vi "ReadNumeric.vi"(1 "reference":refnum<vi>) -> (0 "Numeric":T10)   [LabVIEW 2013]
uses:
  <vilib>/Utility/miscctls.llb/LVBoundsTypeDef.ctl
  <vilib>/Utility/miscctls.llb/LVPositionTypeDef.ctl
  <vilib>/Utility/miscctls.llb/LVRectTypeDef.ctl
  <vilib>/Utility/miscctls.llb/LVDataSocketStatusTypeDef.ctl
  <vilib>/Utility/miscctls.llb/LVKeyNavTypeDef.ctl
  <vilib>/Utility/miscctls.llb/LVMinMaxIncTypeDef.ctl
  <vilib>/Utility/miscctls.llb/LVKeyTypeDef.ctl
  <vilib>/numeric/LVNumericRepresentation.ctl
  <vilib>/Utility/miscctls.llb/LVOutOfRangeActionTypeDef.ctl
panel:
  out "error out 77":errorcluster
  out "error out 76":errorcluster
  out "error out 75":errorcluster
  out "error out 74":errorcluster
  out "error out 73":errorcluster
  out "error out 72":errorcluster
  out "error out 71":errorcluster
  out "error out 70":errorcluster
  out "error out 69":errorcluster
  out "error out 68":errorcluster
  out "error out 67":errorcluster
  out "error out 66":errorcluster
  out "error out 65":errorcluster
  out "error out 64":errorcluster
  out "error out 63":errorcluster
  out "error out 62":errorcluster
  out "error out 61":errorcluster
  out "error out 60":errorcluster
  out "error out 59":errorcluster
  out "error out 58":errorcluster
  out "error out 57":errorcluster
  out "error out 56":errorcluster
  out "error out 55":errorcluster
  out "error out 54":errorcluster
  out "error out 53":errorcluster
  out "error out 52":errorcluster
  out "error out 51":errorcluster
  out "error out 50":errorcluster
  out "error out 49":errorcluster
  out "error out 48":errorcluster
  out "error out 47":errorcluster
  out "error out 46":errorcluster
  out "error out 45":errorcluster
  out "error out 44":errorcluster
  out "error out 43":errorcluster
  out "error out 42":errorcluster
  out "error out 41":errorcluster
  out "error out 40":errorcluster
  out "error out 39":errorcluster
  out "error out 38":errorcluster
  out "error out 37":errorcluster
  out "error out 36":errorcluster
  out "error out 35":errorcluster
  out "error out 34":errorcluster
  out "error out 33":errorcluster
  out "error out 32":errorcluster
  out "error out 31":errorcluster
  out "error out 30":errorcluster
  out "error out 29":errorcluster
  out "error out 28":errorcluster
  out "error out 27":errorcluster
  out "error out 26":errorcluster
  out "error out 25":errorcluster
  out "error out 24":errorcluster
  out "error out 23":errorcluster
  out "error out 22":errorcluster
  out "error out 21":errorcluster
  out "error out 20":errorcluster
  out "error out 19":errorcluster
  out "error out 18":errorcluster
  out "error out 17":errorcluster
  out "error out 16":errorcluster
  out "error out 15":errorcluster
  out "error out 14":errorcluster
  out "error out 13":errorcluster
  out "error out 12":errorcluster
  out "error out 11":errorcluster
  out "error out 10":errorcluster
  out "error out 9":errorcluster
  out "error out 8":errorcluster
  out "error out 7":errorcluster
  out "error out 6":errorcluster
  out "error out 5":errorcluster
  out "error out 4":errorcluster
  out "error out 3":errorcluster
  out "error out 2":errorcluster
  out "error out":errorcluster
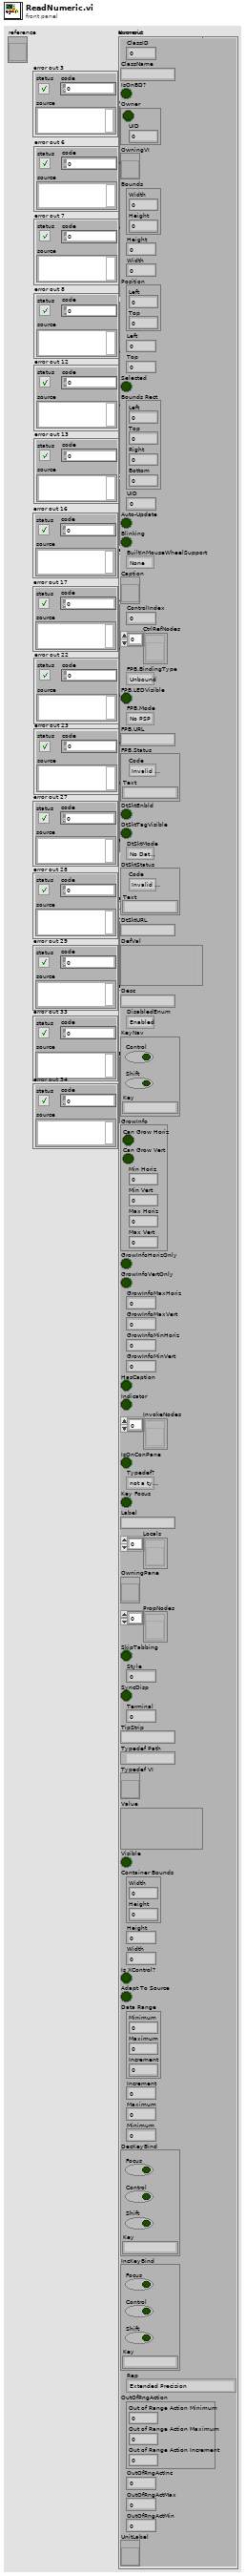
[diagram p1: front panel]
types:
  T1 = typedef "LVBoundsTypeDef.ctl" = cluster{"Width":u32, "Height":u32}
  T2 = typedef "LVPositionTypeDef.ctl" = cluster{"Left":i32, "Top":i32}
  T3 = typedef "LVRectTypeDef.ctl" = cluster{"Left":i16, "Top":i16, "Right":i16, "Bottom":i16}
  T4 = typedef "LVDataSocketStatusTypeDef.ctl" = cluster{"Code":enum32{"Invalid Status", "Unconnected", "Active", "Idle", "Error", "Connecting"}, "Text":string}
  T5 = typedef "LVKeyNavTypeDef.ctl" = cluster{"Control":bool, "Shift":bool, "Key":string}
  T6 = typedef "LVMinMaxIncTypeDef.ctl" = cluster{"Minimum":dbl, "Maximum":dbl, "Increment":dbl}
  T7 = typedef "LVKeyTypeDef.ctl" = cluster{"Focus":bool, "Control":bool, "Shift":bool, "Key":string}
  T8 = typedef "LVNumericRepresentation.ctl" = enum32{"Extended Precision", "Double Precision", "Single Precision", "Long", "Word", "Byte", "Unsigned Long", "Unsigned Word", "Unsigned Byte", "Complex Extended", "Complex Double", "Complex Single", "Quad", "Unsigned Quad", "Fixed-Point"}
  T9 = typedef "LVOutOfRangeActionTypeDef.ctl" = cluster{"Out of Range Action Minimum":u8, "Out of Range Action Maximum":u8, "Out of Range Action Increment":u8}
  T10 = cluster{"ClassID":u32, "ClassName":string, "IsOnBD?":bool, "Owner":cluster{bool, "UID":i32}, "OwningVI":refnum<vi>, "Bounds":T1, "Height":u32, "Width":u32, "Position":T2, "Left":i32, "Top":i32, "Selected":bool, "Bounds Rect":T3, "UID":i32, "Auto-Update":bool, "Blinking":bool, "BuiltInMouseWheelSupport":enum16{"None", "On Hover", "On Key Focus", "On Hover or Key Focus"}, "Caption":refnum<vi>, "ControlIndex":i32, "CtrlRefNodes":refnum<vi>[], "FPB.BindingType":enum32{"Unbound", "Bound To PSP URL", "Bound To Variable Shortcut"}, "FPB.LEDVisible":bool, "FPB.Mode":enum32{"No PSP", "Read", "Write", "Write & Read"}, "FPB.URL":string, "FPB.Status":T4, "DtSktEnbld":bool, "DtSktTagVisible":bool, "DtSktMode":enum32{"No DataSocket", "Publish", "Subscribe", "Publish & Subscribe"}, "DtSktStatus":T4, "DtSktURL":string, "DefVal":variant, "Desc":string, "DisabledEnum":enum8{"Enabled", "Disabled", "Disabled and Grayed Out"}, "KeyNav":T5, "GrowInfo":cluster{"Can Grow Horiz":bool, "Can Grow Vert":bool, "Min Horiz":i16, "Min Vert":i16, "Max Horiz":i16, "Max Vert":i16}, "GrowInfoHorizOnly":bool, "GrowInfoVertOnly":bool, "GrowInfoMaxHoriz":i16, "GrowInfoMaxVert":i16, "GrowInfoMinHoriz":i16, "GrowInfoMinVert":i16, "HasCaption":bool, "Indicator":bool, "InvokeNodes":refnum<vi>[], "IsOnConPane":bool, "Typedef?":enum32{"not a typedef", "typedef", "strict typedef", "class private data"}, "Key Focus":bool, "Label":string, "Locals":refnum<vi>[], "OwningPane":refnum<vi>, "PropNodes":refnum<vi>[], "SkipTabbing":bool, "Style":u32, "SyncDisp":bool, "Terminal":i32, "TipStrip":string, "Typedef Path":path, "Typedef VI":refnum<vi>, "Value":variant, "Visible":bool, "Container Bounds":T1, "Height":u32, "Width":u32, "Is XControl?":bool, "Adapt To Source":bool, "Data Range":T6, "Increment":dbl, "Maximum":dbl, "Minimum":dbl, "DecKeyBind":T7, "IncKeyBind":T7, "Rep":T8, "OutOfRngAction":T9, "OutOfRngActInc":u8, "OutOfRngActMax":u8, "OutOfRngActMin":u8, "UnitLabel":refnum<vi>}
  T11 = enum16{"None", "On Hover", "On Key Focus", "On Hover or Key Focus"}
  T12 = enum32{"No PSP", "Read", "Write", "Write & Read"}
  T13 = enum32{"Unbound", "Bound To PSP URL", "Bound To Variable Shortcut"}
  T14 = enum32{"No DataSocket", "Publish", "Subscribe", "Publish & Subscribe"}
  T15 = enum8{"Enabled", "Disabled", "Disabled and Grayed Out"}
  T16 = enum32{"not a typedef", "typedef", "strict typedef", "class private data"}
  T17 = cluster{"Can Grow Horiz":bool, "Can Grow Vert":bool, "Min Horiz":i16, "Min Vert":i16, "Max Horiz":i16, "Max Vert":i16}
  T18 = cluster{"ClassID":u32, "ClassName":string, "IsOnBD?":bool, "Cluster":cluster{bool, "UID":i32}, "OwningVI":refnum<vi>, "Bounds":T1, "Height":u32, "Width":u32, "Position":T2, "Left":i32, "Top":i32, "Selected":bool, "Bounds Rect":T3, "UID":i32, "Auto-Update":bool, "Blinking":bool, "BuiltInMouseWheelSupport":enum16{"None", "On Hover", "On Key Focus", "On Hover or Key Focus"}, "Caption":refnum<vi>, "ControlIndex":i32, "CtrlRefNodes":refnum<vi>[], "FPB.BindingType":enum32{"Unbound", "Bound To PSP URL", "Bound To Variable Shortcut"}, "FPB.LEDVisible":bool, "FPB.Mode":enum32{"No PSP", "Read", "Write", "Write & Read"}, "FPB.URL":string, "FPB.Status":T4, "DtSktEnbld":bool, "DtSktTagVisible":bool, "DtSktMode":enum32{"No DataSocket", "Publish", "Subscribe", "Publish & Subscribe"}, "DtSktStatus":T4, "DtSktURL":string, "DefVal":variant, "Desc":string, "DisabledEnum":enum8{"Enabled", "Disabled", "Disabled and Grayed Out"}, "KeyNav":T5, "GrowInfo":cluster{"Can Grow Horiz":bool, "Can Grow Vert":bool, "Min Horiz":i16, "Min Vert":i16, "Max Horiz":i16, "Max Vert":i16}, "GrowInfoHorizOnly":bool, "GrowInfoVertOnly":bool, "GrowInfoMaxHoriz":i16, "GrowInfoMaxVert":i16, "GrowInfoMinHoriz":i16, "GrowInfoMinVert":i16, "HasCaption":bool, "Indicator":bool, "InvokeNodes":refnum<vi>[], "IsOnConPane":bool, "Typedef?":enum32{"not a typedef", "typedef", "strict typedef", "class private data"}, "Key Focus":bool, "Text":string, "Locals":refnum<vi>[], "OwningPane":refnum<vi>, "PropNodes":refnum<vi>[], "SkipTabbing":bool, "Style":u32, "SyncDisp":bool, "UID":i32, "TipStrip":string, "Typedef Path":path, "Typedef VI":refnum<vi>, "Value":variant, "Visible":bool, "Container Bounds":T1, "Height":u32, "Width":u32, "Is XControl?":bool, "Adapt To Source":bool, "Data Range":T6, "Increment":dbl, "Maximum":dbl, "Minimum":dbl, "DecKeyBind":T7, "IncKeyBind":T7, "Rep":T8, "OutOfRngAction":T9, "OutOfRngActInc":u8, "OutOfRngActMax":u8, "OutOfRngActMin":u8, "UnitLabel":refnum<vi>}
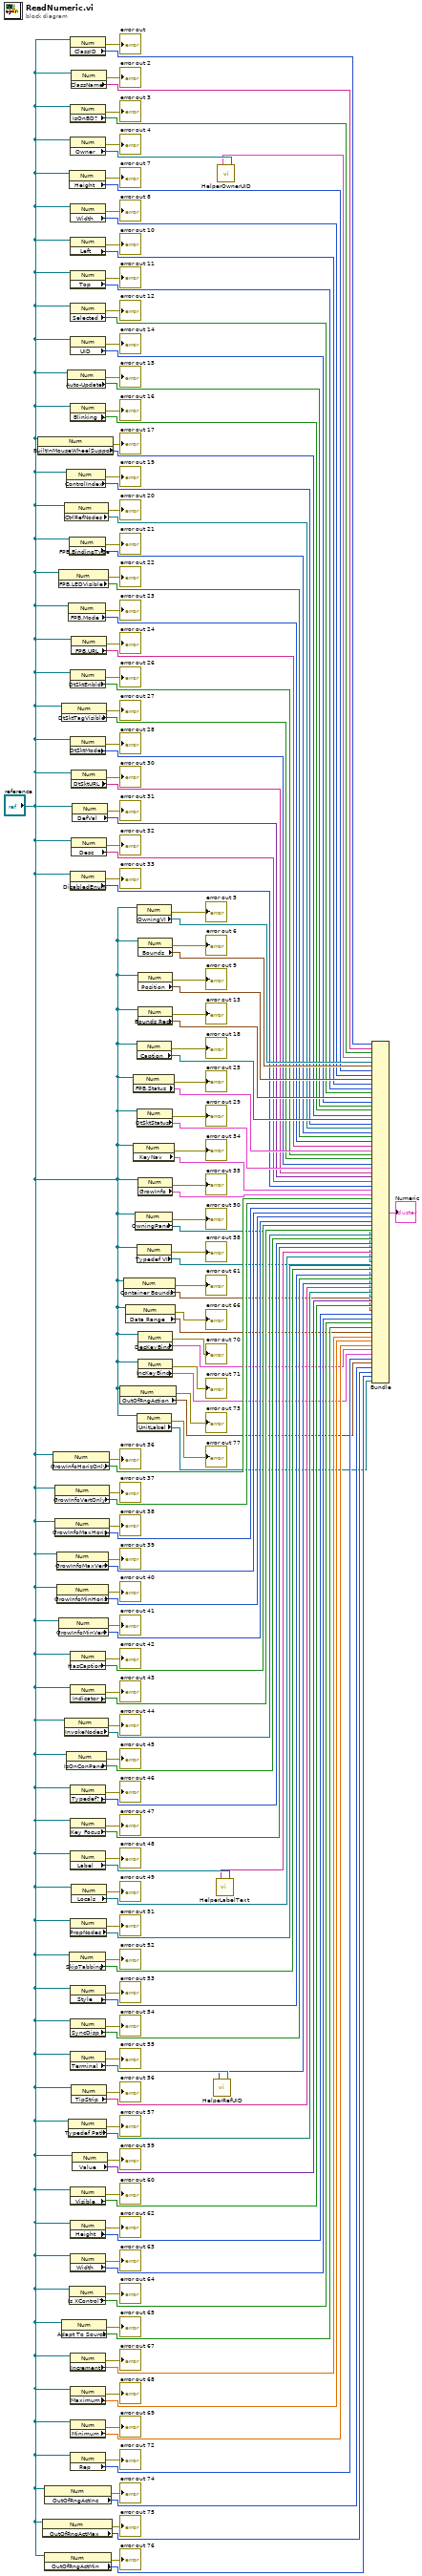
[diagram p0: block diagram]
diagram:
  n1 = property class="Num"(reference="reference") -> (error out=→"error out 17":errorcluster, "BuiltInMouseWheelSupport"=w124:T11)  [unwired: 1 in, 1 out]
  n2 = property class="Num"(reference="reference") -> (error out=→"error out 75":errorcluster, "OutOfRngActMax"=w6:u8)  [unwired: 1 in, 1 out]
  n3 = property class="Num"(reference="reference") -> (error out=→"error out 74":errorcluster, "OutOfRngActInc"=w8:u8)  [unwired: 1 in, 1 out]
  n4 = property class="Num"(reference="reference") -> (error out=→"error out 76":errorcluster, "OutOfRngActMin"=w4:u8)  [unwired: 1 in, 1 out]
  n5 = property class="Num"(reference="reference") -> (error out=→"error out 36":errorcluster, "GrowInfoHorizOnly"=w86:bool)  [unwired: 1 in, 1 out]
  n6 = property class="Num"(reference="reference") -> (error out=→"error out 37":errorcluster, "GrowInfoVertOnly"=w84:bool)  [unwired: 1 in, 1 out]
  n7 = property class="Num"(reference="reference") -> (error out=→"error out 38":errorcluster, "GrowInfoMaxHoriz"=w82:i16)  [unwired: 1 in, 1 out]
  n8 = property class="Num"(reference="reference") -> (error out=→"error out 39":errorcluster, "GrowInfoMaxVert"=w80:i16)  [unwired: 1 in, 1 out]
  n9 = property class="Num"(reference="reference") -> (error out=→"error out 40":errorcluster, "GrowInfoMinHoriz"=w78:i16)  [unwired: 1 in, 1 out]
  n10 = property class="Num"(reference="reference") -> (error out=→"error out 22":errorcluster, "FPB.LEDVisible"=w114:bool)  [unwired: 1 in, 1 out]
  n11 = property class="Num"(reference="reference") -> (error out=→"error out 41":errorcluster, "GrowInfoMinVert"=w76:i16)  [unwired: 1 in, 1 out]
  n12 = property class="Num"(reference="reference") -> (error out=→"error out 27":errorcluster, "DtSktTagVisible"=w104:bool)  [unwired: 1 in, 1 out]
  n13 = property class="Num"(reference="reference") -> (error out=→"error out 65":errorcluster, "Adapt To Source"=w26:bool)  [unwired: 1 in, 1 out]
  n14 = property class="Num"(reference="reference") -> (error out=→"error out 20":errorcluster, "CtrlRefNodes"=w118:refnum<vi>[])  [unwired: 1 in, 1 out]
  n15 = property class="Num"(reference="reference") -> (error out=→"error out 44":errorcluster, "InvokeNodes"=w70:refnum<vi>[])  [unwired: 1 in, 1 out]
  n16 = property class="Num"(reference="reference") -> (error out=→"error out 45":errorcluster, "IsOnConPane"=w68:bool)  [unwired: 1 in, 1 out]
  n17 = property class="Num"(reference="reference") -> (error out=→"error out 19":errorcluster, "ControlIndex"=w120:i32)  [unwired: 1 in, 1 out]
  n18 = property class="Num"(reference="reference") -> (error out=→"error out 15":errorcluster, "Auto-Update"=w128:bool)  [unwired: 1 in, 1 out]
  n19 = property class="Num"(reference="reference") -> (error out=→"error out 23":errorcluster, "FPB.Mode"=w112:T12)  [unwired: 1 in, 1 out]
  n20 = property class="Num"(reference="reference") -> (error out=→"error out 57":errorcluster, "Typedef Path"=w42:path)  [unwired: 1 in, 1 out]
  n21 = property class="Num"(reference="reference") -> (error out=→"error out 7":errorcluster, "Height"=w144:u32)  [unwired: 1 in, 1 out]
  n22 = property class="Num"(reference="reference") -> (error out=→"error out 21":errorcluster, "FPB.BindingType"=w116:T13)  [unwired: 1 in, 1 out]
  n23 = property class="Num"(reference="reference") -> (error out=→"error out 52":errorcluster, "SkipTabbing"=w53:bool)  [unwired: 1 in, 1 out]
  n24 = property class="Num"(reference="reference") -> (error out=→"error out 64":errorcluster, "Is XControl?"=w28:bool)  [unwired: 1 in, 1 out]
  n25 = property class="Num"(reference="reference") -> (error out=→"error out 51":errorcluster, "PropNodes"=w55:refnum<vi>[])  [unwired: 1 in, 1 out]
  n26 = property class="Num"(reference="reference") -> (error out=→"error out":errorcluster, "ClassID"=w157:u32)  [unwired: 1 in, 1 out]
  n27 = property class="Num"(reference="reference") -> (error out=→"error out 3":errorcluster, "IsOnBD?"=w153:bool)  [unwired: 1 in, 1 out]
  n28 = property class="Num"(reference="reference") -> (error out=→"error out 4":errorcluster, "Owner"=w151:refnum<vi>)  [unwired: 1 in, 1 out]
  n29 = property class="Num"(reference="reference") -> (error out=→"error out 8":errorcluster, "Width"=w142:u32)  [unwired: 1 in, 1 out]
  n30 = property class="Num"(reference="reference") -> (error out=→"error out 10":errorcluster, "Left"=w138:i32)  [unwired: 1 in, 1 out]
  n31 = property class="Num"(reference="reference") -> (error out=→"error out 11":errorcluster, "Top"=w136:i32)  [unwired: 1 in, 1 out]
  n32 = property class="Num"(reference="reference") -> (error out=→"error out 12":errorcluster, "Selected"=w134:bool)  [unwired: 1 in, 1 out]
  n33 = property class="Num"(reference="reference") -> (error out=→"error out 14":errorcluster, "UID"=w130:i32)  [unwired: 1 in, 1 out]
  n34 = property class="Num"(reference="reference") -> (error out=→"error out 16":errorcluster, "Blinking"=w126:bool)  [unwired: 1 in, 1 out]
  n35 = property class="Num"(reference="reference") -> (error out=→"error out 26":errorcluster, "DtSktEnbld"=w106:bool)  [unwired: 1 in, 1 out]
  n36 = property class="Num"(reference="reference") -> (error out=→"error out 28":errorcluster, "DtSktMode"=w102:T14)  [unwired: 1 in, 1 out]
  n37 = property class="Num"(reference="reference") -> (error out=→"error out 33":errorcluster, "DisabledEnum"=w92:T15)  [unwired: 1 in, 1 out]
  n38 = property class="Num"(reference="reference") -> (error out=→"error out 42":errorcluster, "HasCaption"=w74:bool)  [unwired: 1 in, 1 out]
  n39 = property class="Num"(reference="reference") -> (error out=→"error out 43":errorcluster, "Indicator"=w72:bool)  [unwired: 1 in, 1 out]
  n40 = property class="Num"(reference="reference") -> (error out=→"error out 46":errorcluster, "Typedef?"=w66:T16)  [unwired: 1 in, 1 out]
  n41 = property class="Num"(reference="reference") -> (error out=→"error out 47":errorcluster, "Key Focus"=w64:bool)  [unwired: 1 in, 1 out]
  n42 = property class="Num"(reference="reference") -> (error out=→"error out 48":errorcluster, "Label"=w62:refnum<vi>)  [unwired: 1 in, 1 out]
  n43 = property class="Num"(reference="reference") -> (error out=→"error out 53":errorcluster, "Style"=w51:u32)  [unwired: 1 in, 1 out]
  n44 = property class="Num"(reference="reference") -> (error out=→"error out 54":errorcluster, "SyncDisp"=w49:bool)  [unwired: 1 in, 1 out]
  n45 = property class="Num"(reference="reference") -> (error out=→"error out 55":errorcluster, "Terminal"=w47:refnum<vi>)  [unwired: 1 in, 1 out]
  n46 = property class="Num"(reference="reference") -> (error out=→"error out 60":errorcluster, "Visible"=w36:bool)  [unwired: 1 in, 1 out]
  n47 = property class="Num"(reference="reference") -> (error out=→"error out 62":errorcluster, "Height"=w32:u32)  [unwired: 1 in, 1 out]
  n48 = property class="Num"(reference="reference") -> (error out=→"error out 63":errorcluster, "Width"=w30:u32)  [unwired: 1 in, 1 out]
  n49 = property class="Num"(reference="reference") -> (error out=→"error out 67":errorcluster, "Increment"=w22:dbl)  [unwired: 1 in, 1 out]
  n50 = property class="Num"(reference="reference") -> (error out=→"error out 68":errorcluster, "Maximum"=w20:dbl)  [unwired: 1 in, 1 out]
  n51 = property class="Num"(reference="reference") -> (error out=→"error out 69":errorcluster, "Minimum"=w18:dbl)  [unwired: 1 in, 1 out]
  n52 = property class="Num"(reference="reference") -> (error out=→"error out 72":errorcluster, "Rep"=w12:T8)  [unwired: 1 in, 1 out]
  n53 = property class="Num"(reference="reference") -> (error out=→"error out 2":errorcluster, "ClassName"=w155:string)  [unwired: 1 in, 1 out]
  n54 = property class="Num"(reference="reference") -> (error out=→"error out 24":errorcluster, "FPB.URL"=w110:string)  [unwired: 1 in, 1 out]
  n55 = property class="Num"(reference="reference") -> (error out=→"error out 30":errorcluster, "DtSktURL"=w98:string)  [unwired: 1 in, 1 out]
  n56 = property class="Num"(reference="reference") -> (error out=→"error out 32":errorcluster, "Desc"=w94:string)  [unwired: 1 in, 1 out]
  n57 = property class="Num"(reference="reference") -> (error out=→"error out 49":errorcluster, "Locals"=w59:refnum<vi>[])  [unwired: 1 in, 1 out]
  n58 = property class="Num"(reference="reference") -> (error out=→"error out 56":errorcluster, "TipStrip"=w44:string)  [unwired: 1 in, 1 out]
  n59 = property class="Num"(reference="reference") -> (error out=→"error out 31":errorcluster, "DefVal"=w96:variant)  [unwired: 1 in, 1 out]
  n60 = property class="Num"(reference="reference") -> (error out=→"error out 59":errorcluster, "Value"=w38:variant)  [unwired: 1 in, 1 out]
  n61 = property class="Num"(reference="reference") -> (error out=→"error out 73":errorcluster, "OutOfRngAction"=w10:T9)  [unwired: 1 in, 1 out]
  n62 = property class="Num"(reference="reference") -> (error out=→"error out 61":errorcluster, "Container Bounds"=w34:T1)  [unwired: 1 in, 1 out]
  n63 = property class="Num"(reference="reference") -> (error out=→"error out 66":errorcluster, "Data Range"=w24:T6)  [unwired: 1 in, 1 out]
  n64 = property class="Num"(reference="reference") -> (error out=→"error out 25":errorcluster, "FPB.Status"=w108:T4)  [unwired: 1 in, 1 out]
  n65 = property class="Num"(reference="reference") -> (error out=→"error out 34":errorcluster, "KeyNav"=w90:T5)  [unwired: 1 in, 1 out]
  n66 = property class="Num"(reference="reference") -> (error out=→"error out 50":errorcluster, "OwningPane"=w57:refnum<vi>)  [unwired: 1 in, 1 out]
  n67 = property class="Num"(reference="reference") -> (error out=→"error out 5":errorcluster, "OwningVI"=w148:refnum<vi>)  [unwired: 1 in, 1 out]
  n68 = property class="Num"(reference="reference") -> (error out=→"error out 18":errorcluster, "Caption"=w122:refnum<vi>)  [unwired: 1 in, 1 out]
  n69 = property class="Num"(reference="reference") -> (error out=→"error out 29":errorcluster, "DtSktStatus"=w100:T4)  [unwired: 1 in, 1 out]
  n70 = property class="Num"(reference="reference") -> (error out=→"error out 58":errorcluster, "Typedef VI"=w40:refnum<vi>)  [unwired: 1 in, 1 out]
  n71 = property class="Num"(reference="reference") -> (error out=→"error out 77":errorcluster, "UnitLabel"=w2:refnum<vi>)  [unwired: 1 in, 1 out]
  n72 = property class="Num"(reference="reference") -> (error out=→"error out 6":errorcluster, "Bounds"=w146:T1)  [unwired: 1 in, 1 out]
  n73 = property class="Num"(reference="reference") -> (error out=→"error out 9":errorcluster, "Position"=w140:T2)  [unwired: 1 in, 1 out]
  n74 = property class="Num"(reference="reference") -> (error out=→"error out 13":errorcluster, "Bounds Rect"=w132:T3)  [unwired: 1 in, 1 out]
  n75 = property class="Num"(reference="reference") -> (error out=→"error out 35":errorcluster, "GrowInfo"=w88:T17)  [unwired: 1 in, 1 out]
  n76 = property class="Num"(reference="reference") -> (error out=→"error out 70":errorcluster, "DecKeyBind"=w16:T7)  [unwired: 1 in, 1 out]
  n77 = property class="Num"(reference="reference") -> (error out=→"error out 71":errorcluster, "IncKeyBind"=w14:T7)  [unwired: 1 in, 1 out]
  n78 = call "HelperRefUID.vi"("Text in"=w47) -> ("UID"=w46:i32)
  n79 = call "HelperLabelText.vi"("Text in"=w62) -> ("Text"=w61:string)
  n80 = call "HelperOwnerUID.vi"("Generic in"=w151) -> ("Cluster"=w150:cluster{bool, "UID":i32})
  n81 = Bundle("ClassID"=w157, "ClassName"=w155, "IsOnBD?"=w153, "Cluster"=w150, "OwningVI"=w148, "Bounds"=w146, "Height"=w144, "Width"=w142, "Position"=w140, "Left"=w138, "Top"=w136, "Selected"=w134, "Bounds Rect"=w132, "UID"=w130, "Auto-Update"=w128, "Blinking"=w126, "BuiltInMouseWheelSupport"=w124, "Caption"=w122, "ControlIndex"=w120, "CtrlRefNodes"=w118, "FPB.BindingType"=w116, "FPB.LEDVisible"=w114, "FPB.Mode"=w112, "FPB.URL"=w110, "FPB.Status"=w108, "DtSktEnbld"=w106, "DtSktTagVisible"=w104, "DtSktMode"=w102, "DtSktStatus"=w100, "DtSktURL"=w98, "DefVal"=w96, "Desc"=w94, "DisabledEnum"=w92, "KeyNav"=w90, "GrowInfo"=w88, "GrowInfoHorizOnly"=w86, "GrowInfoVertOnly"=w84, "GrowInfoMaxHoriz"=w82, "GrowInfoMaxVert"=w80, "GrowInfoMinHoriz"=w78, "GrowInfoMinVert"=w76, "HasCaption"=w74, "Indicator"=w72, "InvokeNodes"=w70, "IsOnConPane"=w68, "Typedef?"=w66, "Key Focus"=w64, "Text"=w61, "Locals"=w59, "OwningPane"=w57, "PropNodes"=w55, "SkipTabbing"=w53, "Style"=w51, "SyncDisp"=w49, "UID"=w46, "TipStrip"=w44, "Typedef Path"=w42, "Typedef VI"=w40, "Value"=w38, "Visible"=w36, "Container Bounds"=w34, "Height"=w32, "Width"=w30, "Is XControl?"=w28, "Adapt To Source"=w26, "Data Range"=w24, "Increment"=w22, "Maximum"=w20, "Minimum"=w18, "DecKeyBind"=w16, "IncKeyBind"=w14, "Rep"=w12, "OutOfRngAction"=w10, "OutOfRngActInc"=w8, "OutOfRngActMax"=w6, "OutOfRngActMin"=w4, "UnitLabel"=w2) -> (→"Numeric":T18)  [unwired: 1 in]
